vi "Load Specific DAC defaults.vi"(8 "error in":errorcluster, 11 "DAC in":refnum<class "DAC.lvclass">) -> (0 "error out":errorcluster, 3 "DAC out":refnum<class "DAC.lvclass">)   [LabVIEW 2019, in "DAC.lvlib" / "DAC.lvclass"]
uses:
  DAC.lvclass
  <vilib>/Utility/error.llb/Error Cluster From Error Code.vi
  <vilib>/ErrorRing/Error Ring.xnode
  <vilib>/Utility/config.llb/NI_LVConfig.lvlib
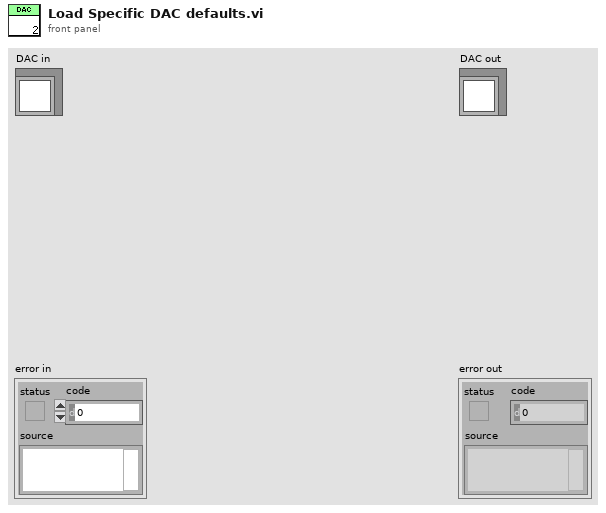
[diagram p1: front panel]
types:
  T1 = typedef "NI_LVConfig.lvlib/Config Data RefNum.ctl" = refnum<k1>
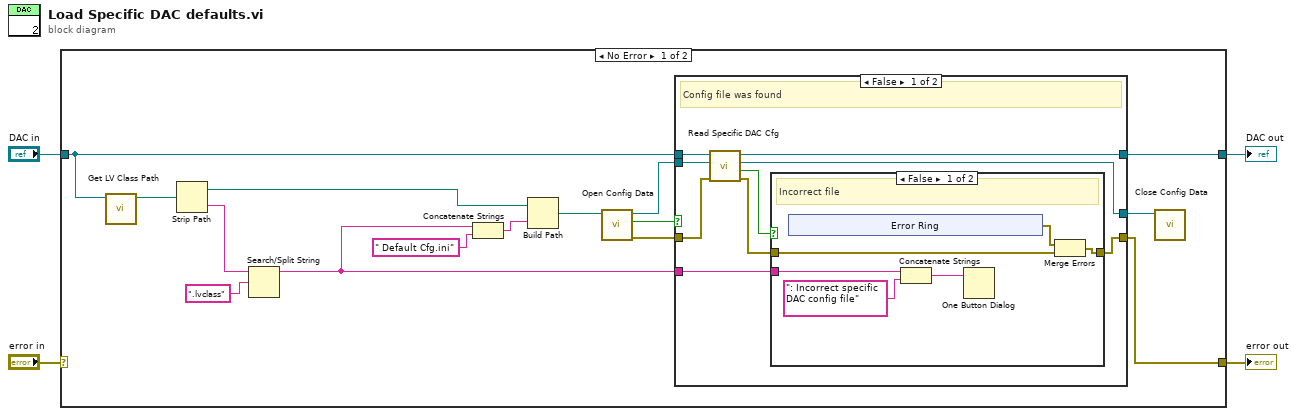
[diagram p0: block diagram]
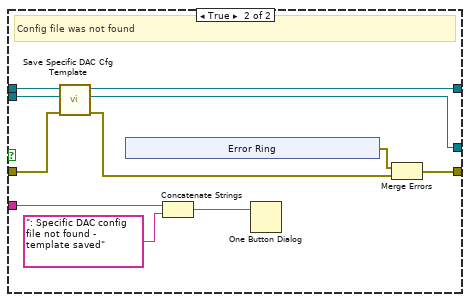
[diagram p3: hidden frame]
diagram:
  n1 = case shown="No Error" "error in" {
    selector: "error in" -> [_ w56]
    tunnel: [w5 w56] -> w3
    tunnel: [w16 w55] -> w1
    tunnel: "DAC in" -> [w17 w55]
    frame No Error {
      n2 = call <vilib>:"Get LV Class Path.vi"("object"=w17) -> ("class path"=w11:path)  [unwired: 9 in, 1 out]
      n3 = Strip Path(path=w11) -> (stripped path=w10:path, name=w9:string)
      n4 = Search/Split String(string=w9, search string/char (-)=".lvclass") -> (substring before match=w6:string)  [unwired: 1 in, 2 out]
      n5 = Concatenate Strings(w6, " Default Cfg.ini" ("name or relative path")) -> (w7:string)
      n6 = Build Path(base path=w10, name or relative path=w7) -> (appended path=w18:path)
      n7 = call <vilib>:"Open Config Data.vi"("configuration file path"=w18) -> ("error out"=w13:errorcluster, "file created?"=w14:bool, "refnum"=w15:T1)  [unwired: 8 in]
      n8 = case shown="False" w14 {
        tunnel: w17 -> [w28 w50]
        tunnel: [w27 w47] -> w16
        tunnel: w15 -> [w26 w49]
        tunnel: w13 -> [w25 w48]
        tunnel: [w23 w45] -> w5
        tunnel: [w21 w43] -> w12
        tunnel: w6 -> [w20 w42]
        frame False {
          # "Config file was found"
          n9 = call-dynamic "Read Specific DAC Cfg.vi"("error in"=w25, "Default Config File Refnum"=w26, "DAC in"=w28) -> ("error out"=w24:errorcluster, "Correct file?"=w22:bool, "refnum out"=w21:T1, "DAC out"=w27:refnum<class "DAC.lvclass">)  [unwired: 5 in]
          n10 = case shown="False" w22 {
            tunnel: w24 -> [w33 w39]
            tunnel: [w32 w39] -> w23
            tunnel: w20 -> [w31 _]
            frame False {
              # "Incorrect file"
              n11 = xnode "Error Ring"() -> ("error out"=w34:errorcluster)
              n12 = Concatenate Strings(w31, ": Incorrect specific DAC config file" ("message")) -> (w29:string)
              n13 = One Button Dialog(message=w29) -> ()  [unwired: 1 in, 1 out]
              n14 = Merge Errors(w34, w33) -> (w32:errorcluster)
            }
            frame True {
              # "Correct file"
            }
          }
        }
        frame True {
          # "Config file was not found"
          n15 = call-dynamic "Save Specific DAC Cfg Template.vi"("error in"=w48, "Default Config File Refnum"=w49, "DAC in"=w50) -> ("error out"=w44:errorcluster, "refnum out"=w43:T1, "DAC out"=w47:refnum<class "DAC.lvclass">)  [unwired: 6 in]
          n16 = xnode "Error Ring"() -> ("error out"=w46:errorcluster)
          n17 = Concatenate Strings(w42, ": Specific DAC config file not found - template saved" ("message")) -> (w40:string)
          n18 = One Button Dialog(message=w40) -> ()  [unwired: 1 in, 1 out]
          n19 = Merge Errors(w46, w44) -> (w45:errorcluster)
        }
      }
      n20 = call <vilib>:"Close Config Data.vi"("refnum"=w12) -> ()  [unwired: 9 in, 2 out]
    }
    frame Error {
    }
  }
  "error out" <- w3
  "DAC out" <- w1
